vi "Remove UI without races.vi"(8 "error in":errorcluster, 10 "user event ref":T1, 11 "sub panel ref in":refnum<vi>) -> (0 "error out":errorcluster, 3 "sub panel ref out":refnum<vi>)   [LabVIEW 2013, in "configuration library.lvlib"]
uses:
  configuration library.lvlib
  <vilib>/CEF_TreeControl/Node/UserEventRef.ctl
  <vilib>/CEF_TreeControl/Controls/EventCluster.ctl
  <vilib>/CEF_TreeControl/NISE_CEF_TreeControl.lvlib
  <vilib>/CEF_TreeControl/Node/NISE_CEF_Node.lvclass
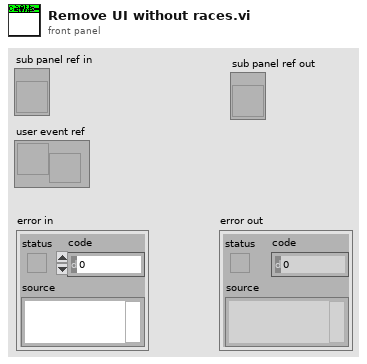
[diagram p1: front panel]
types:
  T1 = typedef "NISE_CEF_Node.lvclass/UserEventRef.ctl" = refnum<user-event>
  T2 = typedef "NISE_CEF_TreeControl.lvlib/EventCluster.ctl" = cluster{"command":string, "data":string}
  T3 = enum32{"Bad", "Idle", "Run top level", "Running"}
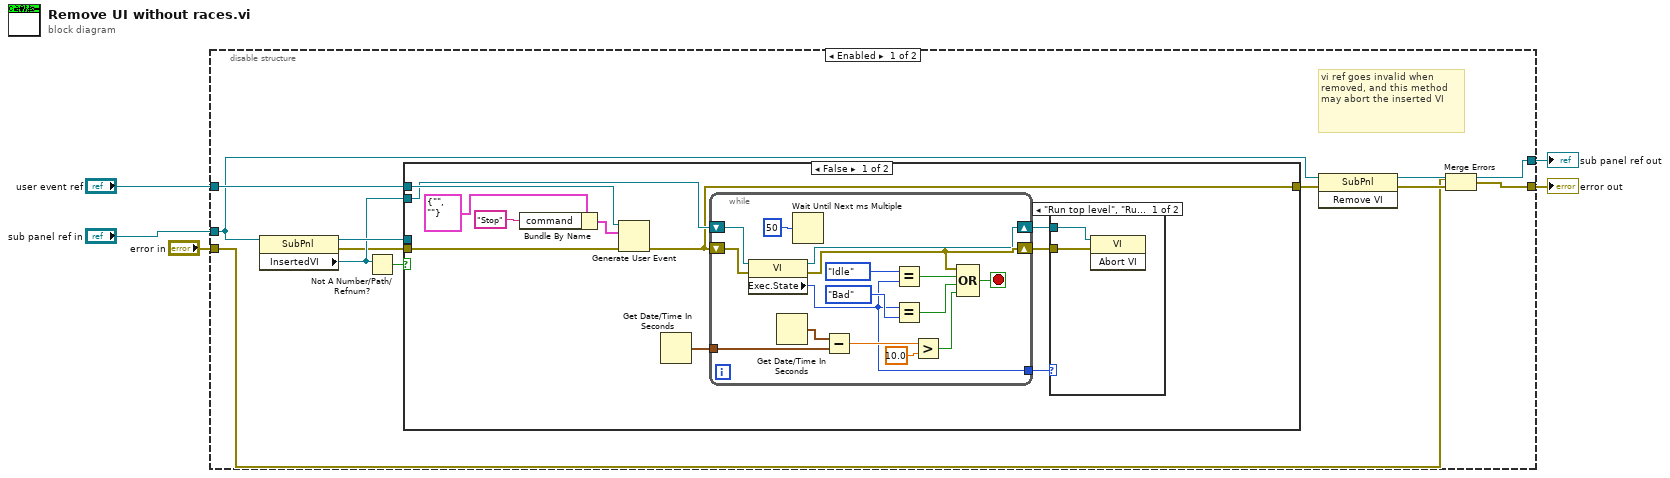
[diagram p0: block diagram]
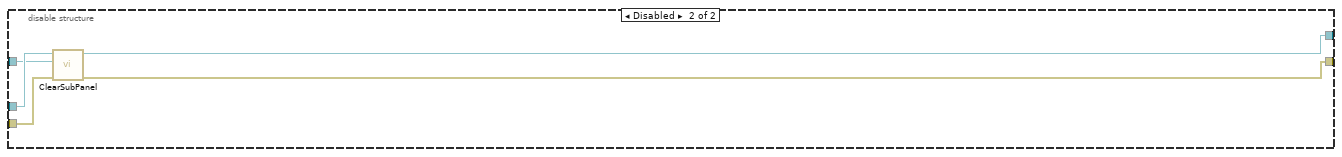
[diagram p4: hidden frame]
diagram:
  n1 = disable-structure shown="Enabled" {
    disable-tunnel: "error in" -> [w9 w51]
    disable-tunnel: "sub panel ref in" -> [w11 w50]
    disable-tunnel: "user event ref" -> [w15 w47]
    disable-tunnel: [w14 w49] -> w2
    disable-tunnel: [w10 w48] -> w1
    frame Enabled {
      # "vi ref goes invalid when removed, and this method may abort the inserted VI"
      n2 = property class="SubPnl"(reference=w11) -> (reference out=w8:refnum<vi>, error out=w6:errorcluster, "InsertedVI"=w7:refnum<vi>)  [unwired: 1 in]
      n3 = Not A Number/Path/Refnum?(number/path/refnum=w7) -> (NaN/Path/Refnum?=w16:bool)
      n4 = case shown="False" w16 {
        tunnel: [w19 w46] -> w13
        tunnel: w7 -> [w22 _]
        tunnel: w6 -> [w17 w46]
        tunnel: w15 -> [w27 _]
        tunnel: w8 -> [_ _]
        frame False {
          n5 = Bundle By Name(cluster=T2 {"command"="", "data"=""} ("event data"), "command"="Stop") -> (w25:T2)
          n6 = Generate User Event(user event=w27, event data cluster=w25, error in=w17) -> (error out=w19:errorcluster)  [unwired: 1 in, 1 out]
          n7 = Get Date/Time In Seconds() -> (seconds since 1Jan1904=w23:timestamp)
          n8 = while {
            tunnel: w23 -> [w42]
            shift-right: [w35] -> w21
            shift-left: w19 -> [w45]
            shift-right: [w31] -> w20
            shift-left: w22 -> [w44]
            tunnel: [w30] -> w18
            stop <- w38 stop-if-true
            n9 = property class="VI"(reference=w44, error in=w45) -> (reference out=w31:refnum<vi>, error out=w35:errorcluster, "Exec.State"=w30:T3)
            n10 = Get Date/Time In Seconds() -> (seconds since 1Jan1904=w43:timestamp)
            n11 = Wait Until Next ms Multiple(millisecond multiple=u32 50 ("milliseconds to wait")) -> ()  [unwired: 1 out]
            n12 = Subtract(x=w43, y=w42) -> (x-y=w41:dbl)
            n13 = Equal?(x=T3."Idle", y=w30) -> (x = y?=w33:bool)
            n14 = Equal?(x=w30, y=T3."Bad") -> (x = y?=w32:bool)
            n15 = Greater?(x=w41, y=10.0) -> (0:w39:bool)
            n16 = Compound Arithmetic op=OR(w35, w33, w32, w39) -> (w38:bool)
          }
          n17 = case shown="\"Run top level\", \"Running\"" w18 {
            tunnel: w21 -> [w29 _]
            tunnel: w20 -> [w28 _]
            frame "Run top level", "Running" {
              n18 = invoke class="VI" method="Abort VI"(reference=w28, error in=w29) -> ()  [unwired: 1 in, 3 out]
            }
            frame "Idle", Default {
            }
          }
        }
        frame True {
          # "Reference is not valid if there is no VI"
        }
      }
      n19 = invoke class="SubPnl" method="Remove VI"(reference=w11, error in=w13) -> (reference out=w14:refnum<vi>, error out=w12:errorcluster)  [unwired: 1 in, 1 out]
      n20 = Merge Errors(w9, w12) -> (w10:errorcluster)
    }
    frame Disabled {
      n21 = call <vilib>:"ClearSubPanel.vi"("error in"=w51, "user event ref"=w47, "sub panel ref in"=w50) -> ("error out"=w48:errorcluster, "sub panel ref out"=w49:refnum<vi>)  [unwired: 7 in]
    }
  }
  "error out" <- w1
  "sub panel ref out" <- w2
